vi "Get_Fast_FID_Calibrations.vi"(1 "Code Name":string, 2 "Calib File String":string, 3 "Take New Data":bool) -> (0 "Calib Constants":dbl[](array[numeric]) format="%.6f")   [LabVIEW 2018]
uses:
  Globals/Meas_global.vi
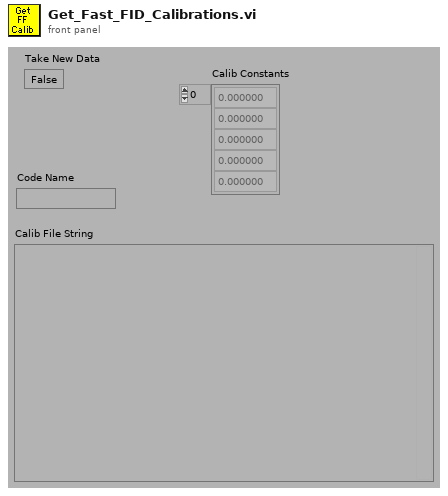
[diagram p1: front panel]
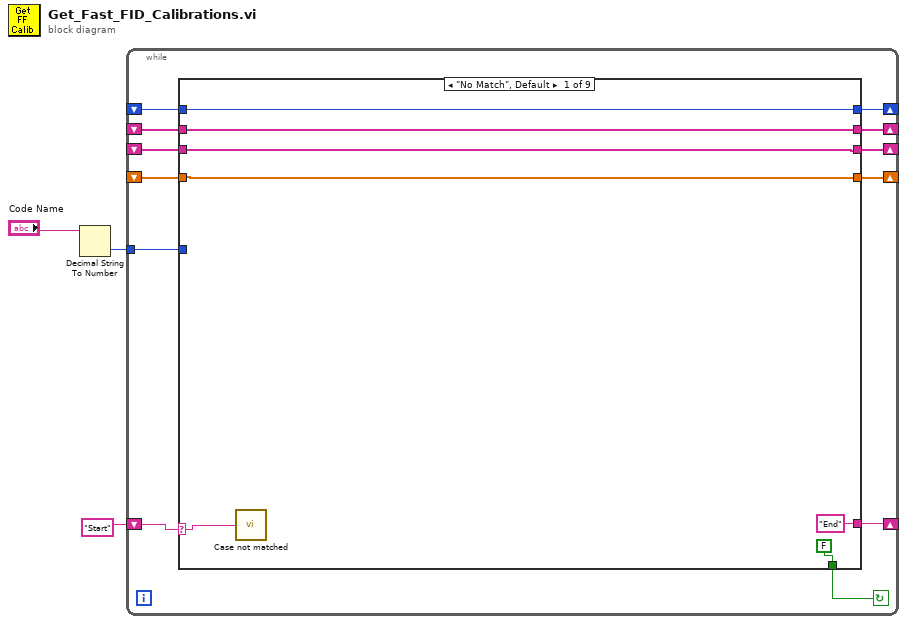
[diagram p0: block diagram]
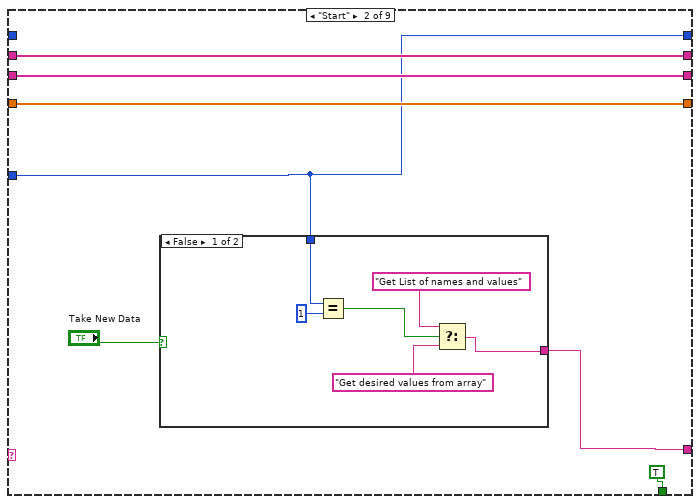
[diagram p2: hidden frame]
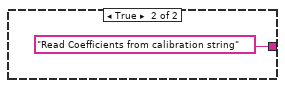
[diagram p3: hidden frame]
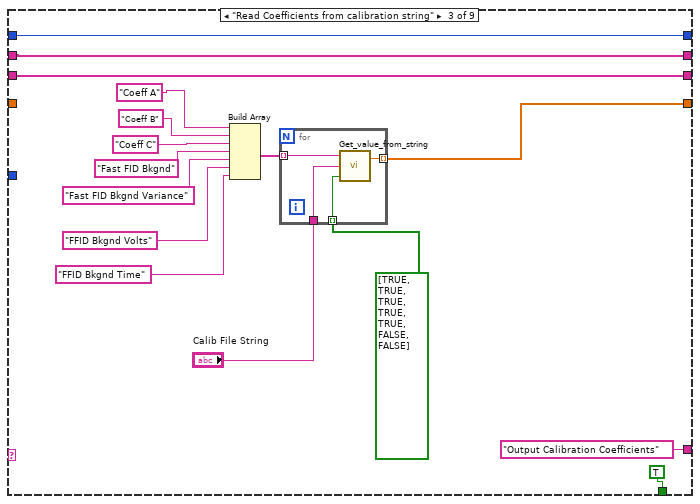
[diagram p4: hidden frame]
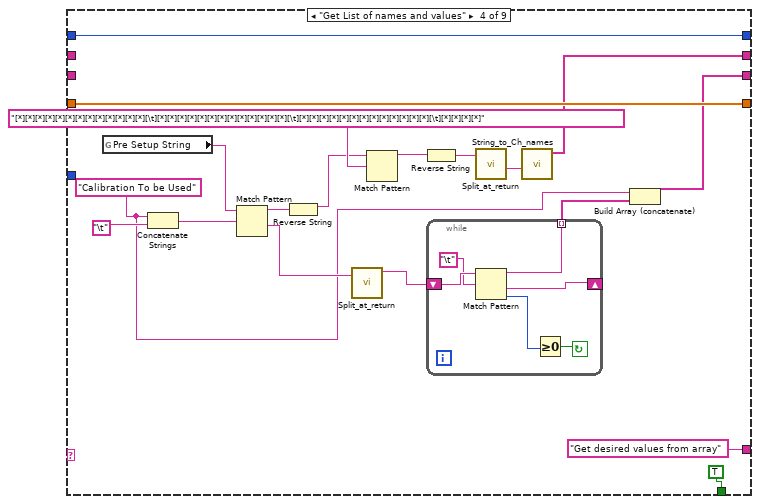
[diagram p5: hidden frame]
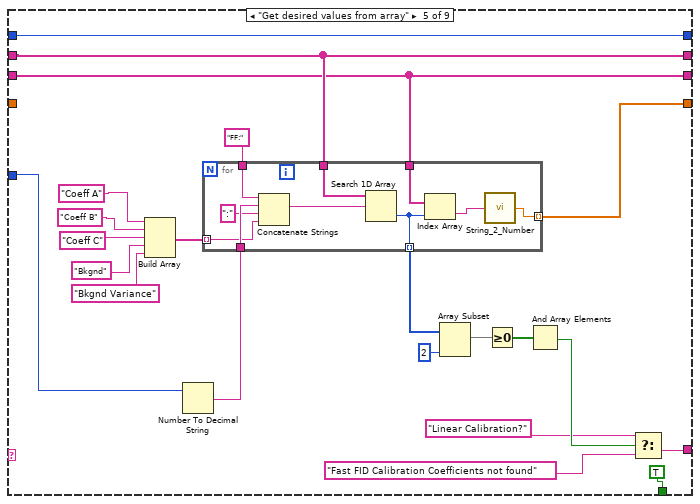
[diagram p6: hidden frame]
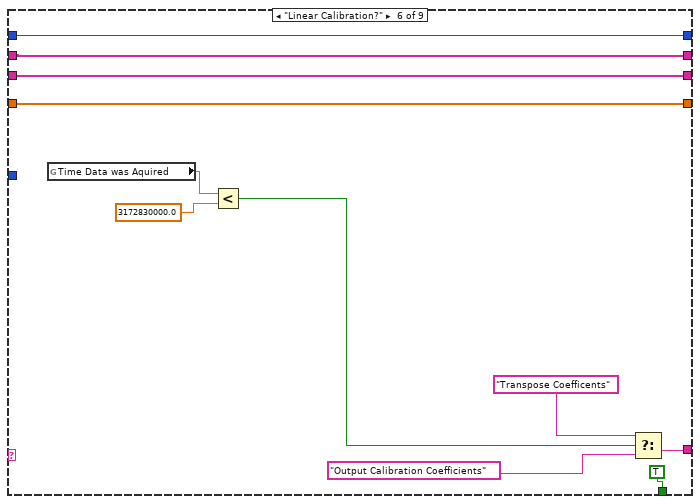
[diagram p7: hidden frame]
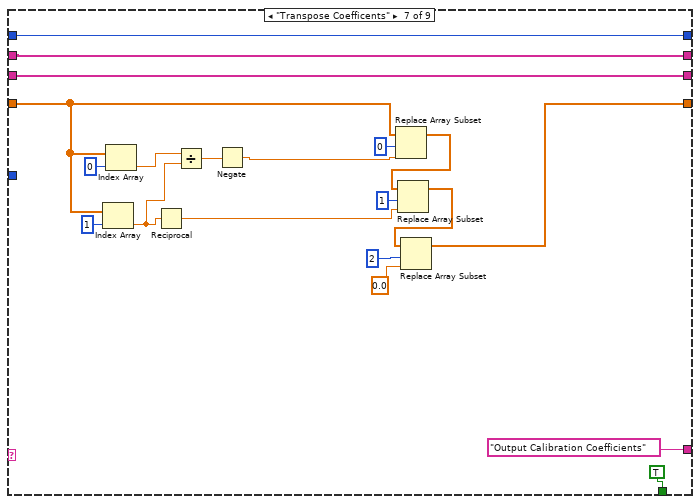
[diagram p8: hidden frame]
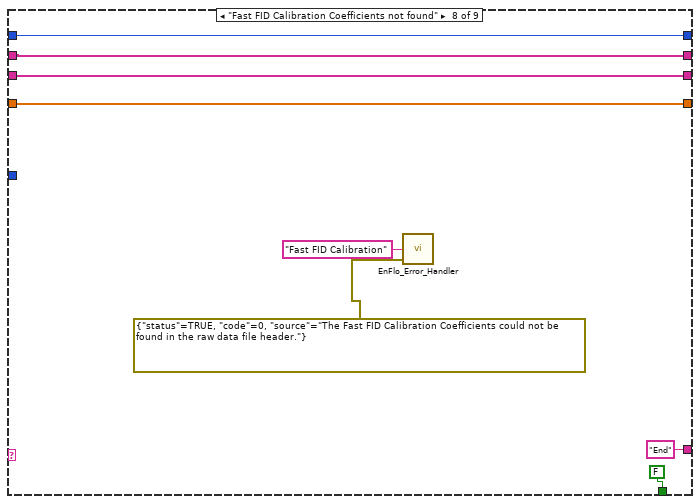
[diagram p9: hidden frame]
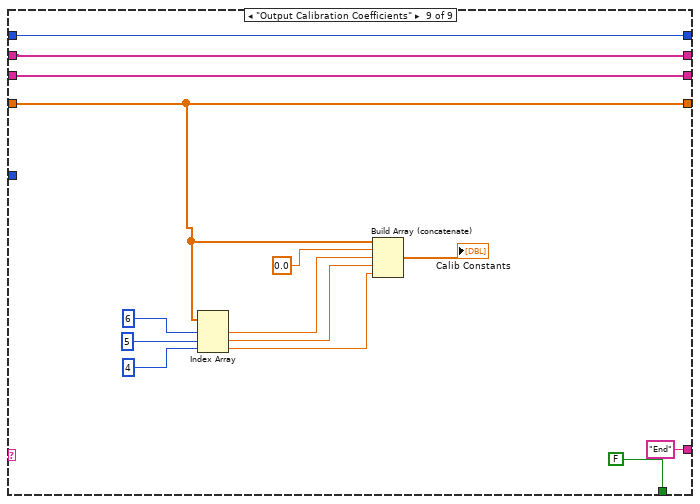
[diagram p10: hidden frame]
diagram:
  n1 = Decimal String To Number(string="Code Name") -> (number=w1:i32)  [unwired: 3 out]
  n2 = while {
    shift-left: _ -> [w10]
    shift-right: [w9] -> _
    shift-left: _ -> [w11]
    shift-right: [w12] -> _
    shift-left: _ -> [w14]
    shift-right: [w13] -> _
    shift-left: "Start" -> [w7]
    shift-right: [w15] -> _
    shift-right: [w6] -> _
    shift-left: _ -> [w5]
    tunnel: w1 -> [w4]
    stop <- w8 continue-if-true
    n3 = case shown="\"No Match\", Default" w7 {
      selector: w7 -> [w16 _ _ _ _ _ _ _ _]
      tunnel: ["End" w26 "Output Calibration Coefficients" "Get desired values from array" w85 w118 "Output Calibration Coefficients" "End" "End"] -> w15
      tunnel: w14 -> [w18 w29 _ w73 _ w114 w134 w145 w159]
      tunnel: [w18 w29 w51 w73 w93 w114 w131 w145 w159] -> w13
      tunnel: w11 -> [w19 w28 w50 _ w94 w121 w141 w149 w165]
      tunnel: [w19 w28 w50 w58 w94 w121 w141 w149 w165] -> w12
      tunnel: w10 -> [w20 _ w49 w75 w102 w123 w143 w151 w164]
      tunnel: [w20 w23 w49 w75 w102 w123 w143 w151 w164] -> w9
      tunnel: [FALSE TRUE TRUE TRUE TRUE TRUE TRUE FALSE FALSE] -> w8
      tunnel: [w17 w24 w48 w62 w95 w122 w142 w150 w162] -> w6
      tunnel: w5 -> [w17 w24 w48 _ w95 w122 w142 w150 w162]
      tunnel: w4 -> [_ w23 _ _ w96 _ _ _ _]
      frame "No Match", Default {
        n4 = call "Case not matched.vi"("Case Name not Matched"=w16) -> ()
      }
      frame "Start" {
        n5 = case shown="False" "Take New Data" {
          tunnel: [w32 "Read Coefficients from calibration string"] -> w26
          tunnel: w23 -> [w35 _]
          frame False {
            n6 = Equal?(x=w35, y=1) -> (x = y?=w33:bool)
            n7 = Select(t="Get List of names and values", s=w33, f="Get desired values from array") -> (s? t:f=w32:string)
          }
          frame True {
          }
        }
      }
      frame "Read Coefficients from calibration string" {
        n8 = Build Array("Coeff A", "Coeff B", "Coeff C", "Fast FID Bkgnd", "Fast FID Bkgnd Variance", "FFID Bkgnd Volts", "FFID Bkgnd Time") -> (w43:string[])
        n9 = for {
          tunnel: w43 -> [w56] mode=indexing
          tunnel: "Calib File String" -> [w55]
          tunnel: [w54] -> w51 mode=indexing
          tunnel: bool[] [TRUE, TRUE, TRUE, TRUE, TRUE, FALSE, FALSE] ("appended array") -> [w53] mode=indexing
          n10 = call "Get_value_from_string.vi"("Show Dialog?"=w53, "Input string"=w55, "Variable name"=w56) -> ("Value"=w54:dbl)  [unwired: 1 out]
        }
      }
      frame "Get List of names and values" {
        w57 = "Calibration To be Used" ("Input Element")
        n11 = global read "Meas_global.vi" "Pre Setup String"() -> (w70:string)
        n12 = Concatenate Strings(w57, "\t") -> (w71:string)
        n13 = Match Pattern(string=w70, regular expression=w71) -> (before substring=w69:string, after substring=w63:string)  [unwired: 3 out]
        n14 = Reverse String(1:w69) -> (0:w67:string)
        n15 = call "Split_at_return.vi"("String"=w63) -> ("before substring"=w74:string)  [unwired: 1 in, 3 out]
        n16 = Match Pattern(string=w67, regular expression="[*][*][*][*][*][*][*][*][*][*][*][*][*][\t][*][*][*][*][*][*][*][*][*][*][*][*][*][\t][*][*][*][*][*][*][*][*][*][*][*][*][*][\t][*][*][*][*]" ("String")) -> (before substring=w66:string)  [unwired: 4 out]
        n17 = Reverse String(1:w66) -> (0:w65:string)
        n18 = while {
          tunnel: [w76] -> w59 mode=indexing
          shift-left: w74 -> [w81]
          shift-right: [w77] -> _
          stop <- w78 continue-if-true
          n19 = Match Pattern(string=w81, regular expression="\t") -> (before substring=w76:string, after substring=w77:string, offset past match=w79:i32)  [unwired: 2 out]
          n20 = Greater Or Equal To 0?(x=w79) -> (x >= 0?=w78:bool)
        }
        n21 = call "Split_at_return.vi"("String"=w65) -> ("after substring"=w64:string)  [unwired: 1 in, 3 out]
        n22 = call "String_to_Ch_names.vi"("Spreadsheet string"=w64) -> ("Ch names"=w62:string[])  [unwired: 3 out]
        n23 = Build Array (concatenate)(w57, w59) -> (w58:string[])
      }
      frame "Get desired values from array" {
        n24 = Build Array("Coeff A", "Coeff B", "Coeff C", "Bkgnd", "Bkgnd Variance") -> (w98:string[])
        n25 = Number To Decimal String(number=w96) -> (decimal integer string=w99:string)  [unwired: 1 out]
        n26 = for {
          tunnel: "FF:" -> [w113]
          tunnel: w99 -> [w112]
          tunnel: w98 -> [w110] mode=indexing
          tunnel: w95 -> [w109]
          tunnel: w94 -> [w107]
          tunnel: [w105] -> w93 mode=indexing
          tunnel: [w104] -> w92 mode=indexing
          n27 = Concatenate Strings(w113, w112, ":" ("Substring"), w110) -> (w108:string)
          n28 = Search 1D Array(1D array=w109, element=w108) -> (index of element=w104:i32)  [unwired: 1 out]
          n29 = Index Array(array=w107, index=w104) -> (element=w106:string)
          n30 = call "String_2_Number.vi"("Value"=w106) -> ("Numeric"=w105:dbl)
        }
        n31 = Array Subset(array=w92, length=2) -> (w90:i32[])  [unwired: 1 in]
        n32 = Greater Or Equal To 0?(x=w90) -> (x >= 0?=w89:bool[])
        n33 = And Array Elements(Boolean array=w89) -> (logical AND=w88:bool)
        n34 = Select(t="Linear Calibration?", s=w88, f="Fast FID Calibration Coefficients not found") -> (s? t:f=w85:string)
      }
      frame "Linear Calibration?" {
        n35 = global read "Meas_global.vi" "Time Data was Aquired"() -> (w117:dbl)
        n36 = Less?(x=w117, y=3172830000.0 ("double precision float")) -> (x < y?=w115:bool)
        n37 = Select(t="Transpose Coefficents", s=w115, f="Output Calibration Coefficients") -> (s? t:f=w118:string)
      }
      frame "Transpose Coefficents" {
        n38 = Index Array(array=w134, index=1) -> (element=w127:dbl)
        n39 = Index Array(array=w134, index=0) -> (element=w128:dbl)
        n40 = Reciprocal(x=w127) -> (1/x=w129:dbl)
        n41 = Divide(x=w128, y=w127) -> (x/y=w126:dbl)
        n42 = Negate(x=w126) -> (-x=w125:dbl)
        n43 = Replace Array Subset(array=w134, new element=w125, index=0) -> (w133:dbl[])
        n44 = Replace Array Subset(array=w133, new element=w129, index=1) -> (w132:dbl[])
        n45 = Replace Array Subset(array=w132, new element=0.0 ("new element/subarray"), index=2) -> (w131:dbl[])
      }
      frame "Fast FID Calibration Coefficients not found" {
        n46 = call "EnFlo_Error_Handler.vi"("error in (no error)"=errorcluster {"status"=TRUE, "code"=0, "source"="The Fast FID Calibration Coefficients could not be found in the raw data file header."}, "Error Type"="Fast FID Calibration") -> ()  [unwired: 1 in, 3 out]
      }
      frame "Output Calibration Coefficients" {
        n47 = Index Array(array=w159, index #1=6 ("index"), index #2=5 ("index"), index #3=4 ("index")) -> (element #1=w155:dbl, element #2=w154:dbl, element #3=w153:dbl)
        n48 = Build Array (concatenate)(w159, 0.0, w155, w154, w153) -> (→"Calib Constants":dbl[])
      }
    }
  }
